vi "Build Method Memory.vi"(8 "Method in":T1, 9 "version":i32, 10 "method":i32, 11 "Method Array in":T1[][](array[typedef])) -> (3 "Method Array out":T1[][](array[typedef]))   [LabVIEW 2012]
uses:
  Method.ctl
panel:
  in  "Empty Method":T1
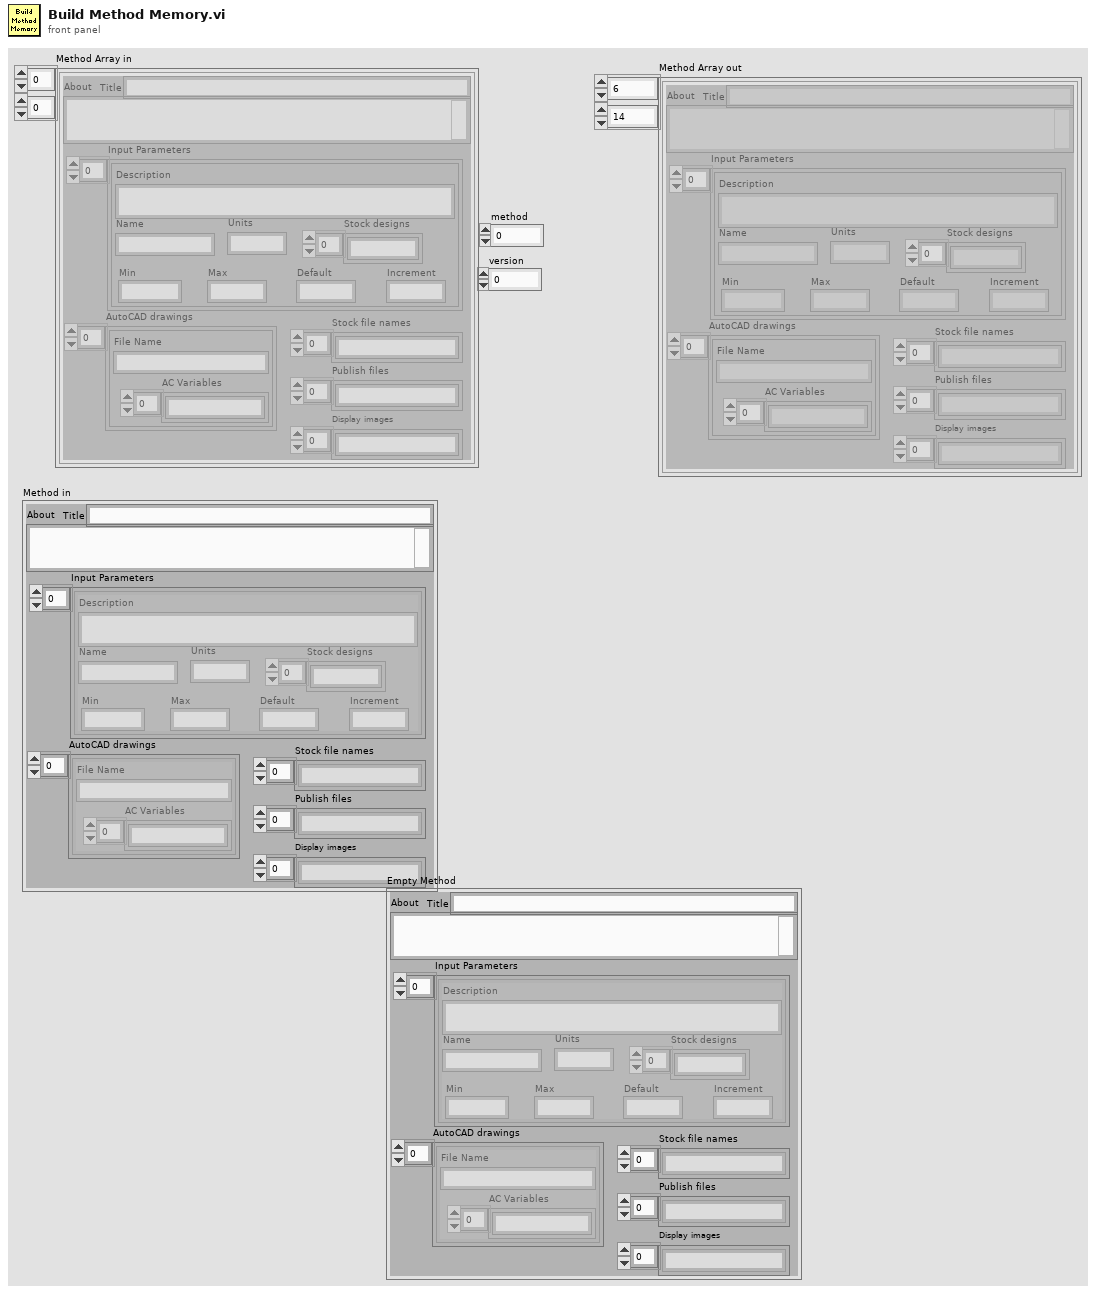
[diagram p1: front panel]
types:
  T1 = typedef "Method.ctl" = cluster{"Title":string, "About":string, "Input Parameters":cluster{"Description":string, "Name":string, "Min":string, "Max":string, "Default":string, "Units":string, "Increment":string, "Stock designs":string[]}[], "AutoCAD drawings":cluster{"File Name":string, "AC Variables":string[]}[], "Stock file names":string[], "Publish files":string[], "Display images":string[]}
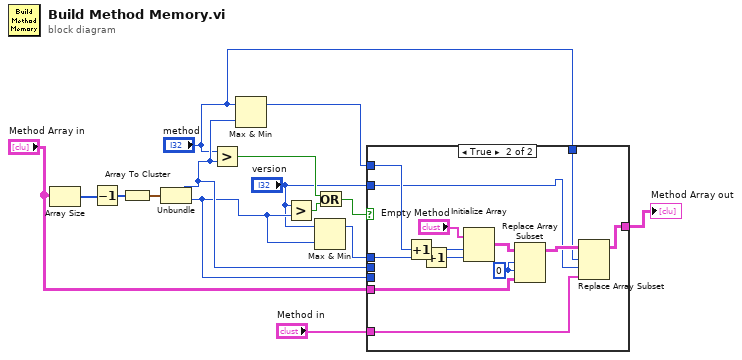
[diagram p0: block diagram]
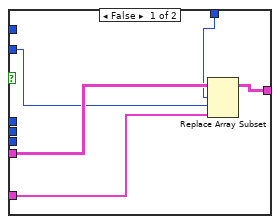
[diagram p2: hidden frame]
diagram:
  n1 = Array Size(array="Method Array in") -> (size(s)=w14:i32[])
  n2 = Decrement(x=w14) -> (x-1=w13:i32[])
  n3 = Array To Cluster(array=w13) -> (cluster=w15:cluster{"[0]":i32, "[1]":i32})
  n4 = Unbundle(w15) -> ("[0]"=w6:i32, "[1]"=w4:i32)
  n5 = Greater?(x="method", y=w6) -> (0:w11:bool)
  n6 = Max & Min(x="method", y=w6) -> (max(x,y)=w5:i32)  [unwired: 1 out]
  n7 = Greater?(x="version", y=w4) -> (0:w12:bool)
  n8 = Max & Min(x="version", y=w4) -> (max(x,y)=w3:i32)  [unwired: 1 out]
  n9 = Or(x=w11, y=w12) -> (x .or. y?=w10:bool)
  n10 = case shown="True" w10 {
    tunnel: w5 -> [_ w32]
    tunnel: w3 -> [_ w31]
    tunnel: "Method Array in" -> [w20 w29]
    tunnel: w6 -> [_ _]
    tunnel: w4 -> [_ _]
    tunnel: "Method in" -> [w19 w27]
    tunnel: [w18 w24] -> w7
    tunnel: "method" -> [w17 w26]
    tunnel: "version" -> [w16 w25]
    frame False {
      n11 = Replace Array Subset(array=w20, new element=w19, index (row)=w17, index (col)=w16) -> (w18:T1[][])
    }
    frame True {
      w21 = 0 ("disabled index (col)")
      n12 = Increment(x=w32) -> (x+1=w23:i32)
      n13 = Increment(x=w31) -> (x+1=w22:i32)
      n14 = Initialize Array("Empty Method", w23, w22) -> (w30:T1[][])
      n15 = Replace Array Subset(array=w30, new element=w29, index (row)=w21, index (col)=w21) -> (w28:T1[][])
      n16 = Replace Array Subset(array=w28, new element=w27, index (row)=w26, index (col)=w25) -> (w24:T1[][])
    }
  }
  "Method Array out" <- w7
